vi "2nd Closest Point.vi"(6 "index to ignore":i32, 8 "line index":i32, 9 "Y in":dbl=359.5 format="%#_13g", 10 "X in":dbl=18.050867335505 format="%#_13g", 11 "All Lines":T1) -> (0 "Index on Line":i32, 3 "Array size":i32)   [LabVIEW 2014]
uses:
  Libraries/Map Data Folder/All-Lines.ctl
  Libraries/Map Data Folder/LineCluster.ctl
  Libraries/Map Data Folder/LineConnection.ctl
  Libraries/Map Data Folder/Map Data.lvlib
panel:
  out "Index found?":bool
  out "Distance to nearest":dbl
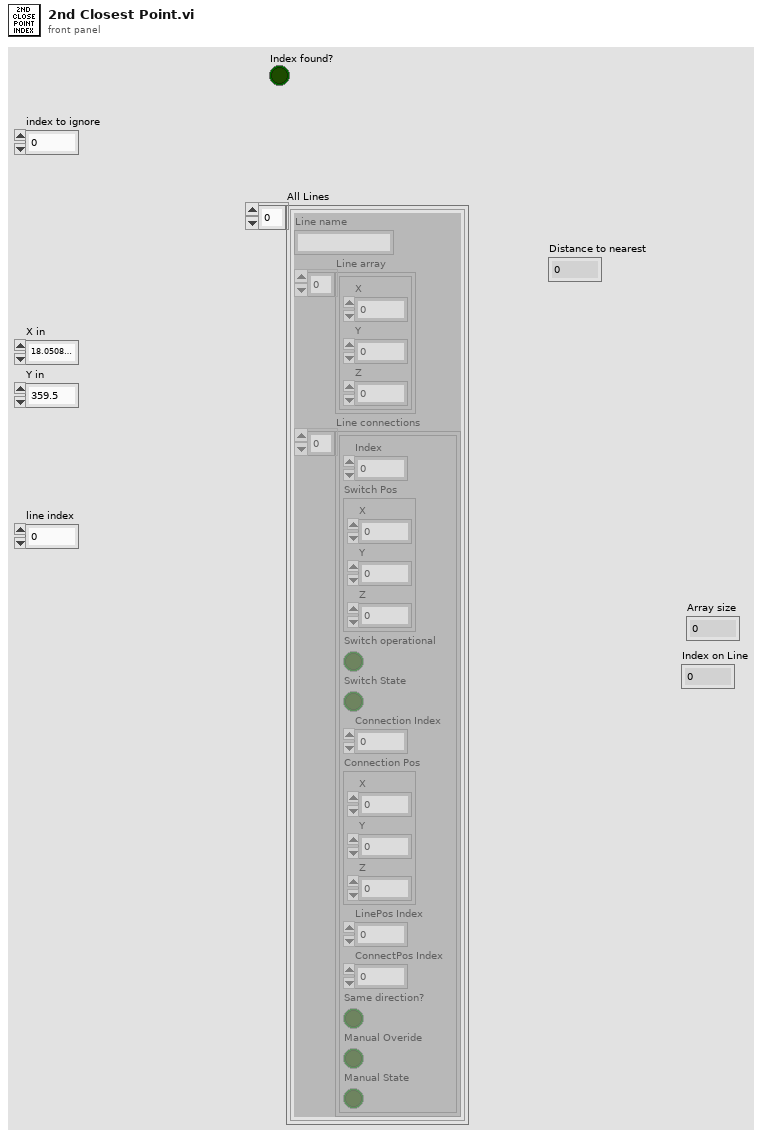
[diagram p1: front panel]
types:
  T1 = typedef "Map Data.lvlib/All-Lines.ctl" = T2[]
  T2 = typedef "Map Data.lvlib/LineCluster.ctl" = cluster{"Line name":string, "Line array":cluster{"X":dbl, "Y":dbl, "Z":dbl}[], "Line connections":T3[]}
  T3 = typedef "Map Data.lvlib/LineConnection.ctl" = cluster{"Index":i32, "Switch Pos":cluster{"X":dbl, "Y":dbl, "Z":dbl}, "Switch operational":bool, "Switch State":bool, "Connection Index":i32, "Connection Pos":cluster{"X":dbl, "Y":dbl, "Z":dbl}, "LinePos Index":i32, "ConnectPos Index":i32, "Same direction?":bool, "Manual Overide":bool, "Manual State":bool}
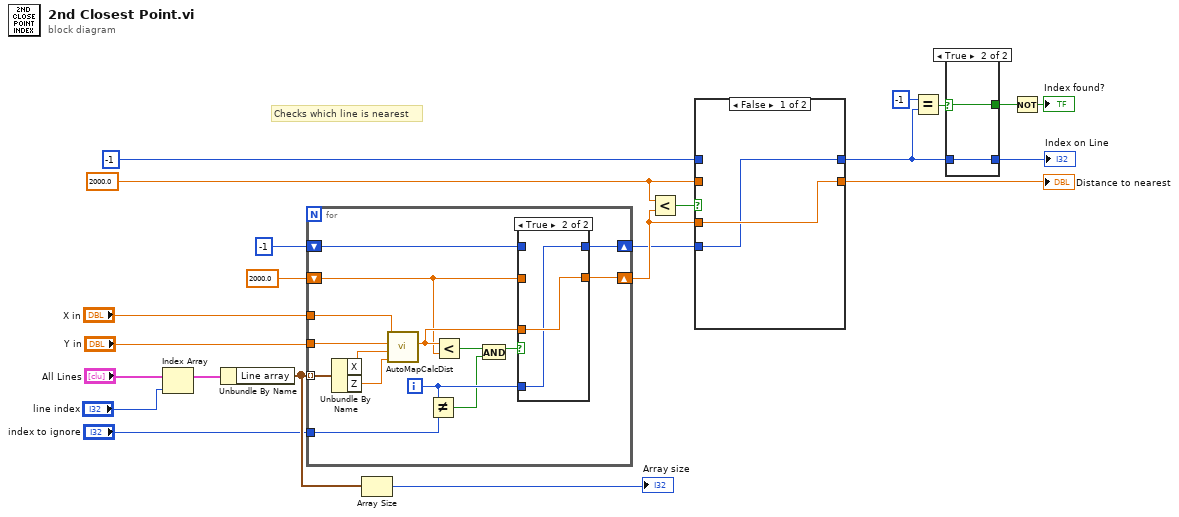
[diagram p0: block diagram]
diagram:
  w21 = 2000.0 ("Distance")
  # "Checks which line is nearest"
  n1 = Index Array(array="All Lines", index="line index") -> (element=w9:T2)
  n2 = Unbundle By Name(w9) -> ("Line array"=w3:cluster{"X":dbl, "Y":dbl, "Z":dbl}[])
  n3 = for {
    tunnel: "X in" -> [w37]
    tunnel: w3 -> [w36] mode=indexing
    tunnel: "Y in" -> [w33]
    shift-right: [w30] -> w13
    shift-left: 2000.0 ("Distance") -> [w31]
    shift-right: [w28] -> w10
    shift-left: -1 -> [w29]
    tunnel: "index to ignore" -> [w25]
    i -> [w26]
    n4 = Unbundle By Name(w36) -> ("X"=w34:dbl, "Z"=w35:dbl)
    n5 = call "AutoMapCalcDist.vi"("Y2"=w35, "X2"=w34, "Y1"=w33, "X1"=w37) -> ("Distance"=w32:dbl)  [unwired: 7 in]
    n6 = Not Equal?(x=w26, y=w25) -> (x != y?=w23:bool)
    n7 = Less?(x=w32, y=w31) -> (x < y?=w27:bool)
    n8 = And(x=w27, y=w23) -> (x .and. y?=w24:bool)
    n9 = case shown="True" w24 {
      tunnel: w32 -> [_ w41]
      tunnel: [w39 w41] -> w30
      tunnel: w31 -> [w39 _]
      tunnel: w29 -> [w38 _]
      tunnel: w26 -> [_ w40]
      tunnel: [w38 w40] -> w28
      frame False {
      }
      frame True {
      }
    }
  }
  n10 = Array Size(array=w3) -> (size(s)=→"Array size":i32)
  n11 = Less?(x=w21, y=w13) -> (x < y?=w12:bool)
  n12 = case shown="False" w12 {
    tunnel: w13 -> [w43 _]
    tunnel: [w43 w45] -> w20
    tunnel: w21 -> [_ w45]
    tunnel: -1 -> [_ w44]
    tunnel: w10 -> [w42 _]
    tunnel: [w42 w44] -> w4
    frame False {
    }
    frame True {
    }
  }
  "Distance to nearest" <- w20
  n13 = Equal?(x=-1, y=w4) -> (x = y?=w15:bool)
  n14 = case shown="True" w15 {
    selector: w15 -> [w46 w49]
    tunnel: [w46 w49] -> w16
    tunnel: w4 -> [w47 w48]
    tunnel: [w47 w48] -> w2
    frame False {
    }
    frame True {
    }
  }
  "Index on Line" <- w2
  n15 = Not(x=w16) -> (.not. x?=→"Index found?":bool)
